vi "test_Bitfile Reload_DMA to Scalar.vi"(8 "error in (no error)":errorcluster, 11 "TestCase in":refnum<class "FPGA Addon Bitfile Reload Unit Tests.lvclass">) -> (0 "error out":errorcluster, 3 "TestCase out":refnum<class "FPGA Addon Bitfile Reload Unit Tests.lvclass">)   [LabVIEW 2020, in "FPGA Addon Bitfile Reload Unit Tests.lvclass"]
uses:
  FPGA Addon Bitfile Reload Unit Tests.lvclass
  APIs/Scripting API/TypeDefs/Output Scalar Data.ctl
  Addon/Addon Shared/Types/FPGA Addon Data Type.ctl
  Addon/Addon Shared/Types/DMA Information.ctl
  Addon/Addon Shared/Types/DMA Settings.ctl
  Addon/Addon Shared/Types/Delacing Scheme.ctl
  Addon/Addon Shared/Types/DMA Acquisition Mode.ctl
  APIs/Scripting API/Public/Bitfile Resources/Import Bitfile Scalars (Instances)/Import Scalars - all.vi
  <vilib>/addons/_JKI Toolkits/VI Tester/TestCase.llb/TestCase.lvclass
  APIs/Scripting API/Scripting API.lvlib
  FPGA Addon Test Class/FPGA Addon Test Class.lvclass
  Addon/Addon System Explorer/FPGA Addon System Explorer.lvlib
  Addon/Addon Shared/FPGA Addon Shared.lvlib
  C:/Program Files (x86)/National Instruments/LabVIEW 2020/vi.lib/addons/_JKI Toolkits/VI Tester/TestCase.llb/TestCase.lvclass
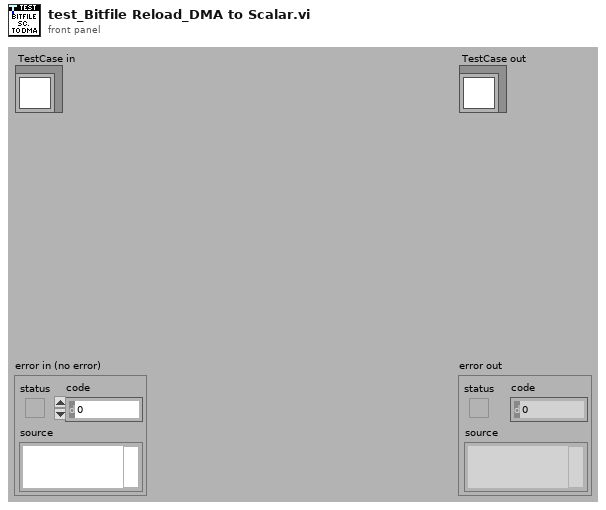
[diagram p1: front panel]
types:
  T1 = typedef "FPGA Addon Shared.lvlib/DMA Information.ctl" = cluster{"Name":string, "Data Type":T2}
  T2 = typedef "FPGA Addon Shared.lvlib/FPGA Addon Data Type.ctl" = enum8{"<Null>", "I8", "I16", "I32", "I64", "U8", "U16", "U32", "U64", "SGL", "Boolean", "Analog PWM In Settings", "Analog PWM In", "Digital PWM In Settings", "Digital PWM In", "Digital PWM Out", "Sine Out", "FXP", "FXP+/-24.5", "FXP+/-16.5", "FXP+/-32.8", "FXP+/-64.32", "FXP+/-16.7", "FXP+/-20.5", "FXP+/-27.5", "FXP+/-32.16", "FXP+16.3", "FXP+18.3", "Digital Static In", "Digital Static Out", "Digital Static In Settings", "Digital WSS Out", "Quad Encoder Settings", "Quad Encoder In", "Group"}
  T3 = typedef "FPGA Addon Shared.lvlib/DMA Settings.ctl" = cluster{"Number of Channels":u8, "Delacing Scheme":T4, "Update Rate":u32, "dt":dbl, "Mode":T5, "Number of Samples":u32, "DMA Host Buffer":u32}
  T4 = typedef "FPGA Addon Shared.lvlib/Delacing Scheme.ctl" = enum8{"Interleaved", "Bitpacked"}
  T5 = typedef "FPGA Addon Shared.lvlib/DMA Acquisition Mode.ctl" = enum8{"Continuous", "Triggered Finite"}
  T6 = typedef "Scripting API.lvlib/Output Scalar Data.ctl" = cluster{"Bitfile Name":string, "SysDef Channel Name":string, "Imported":bool, "Data Type":T2}
  T7 = typedef "Custom Device API.lvlib/Custom Device Item Ref.ctl" = u64
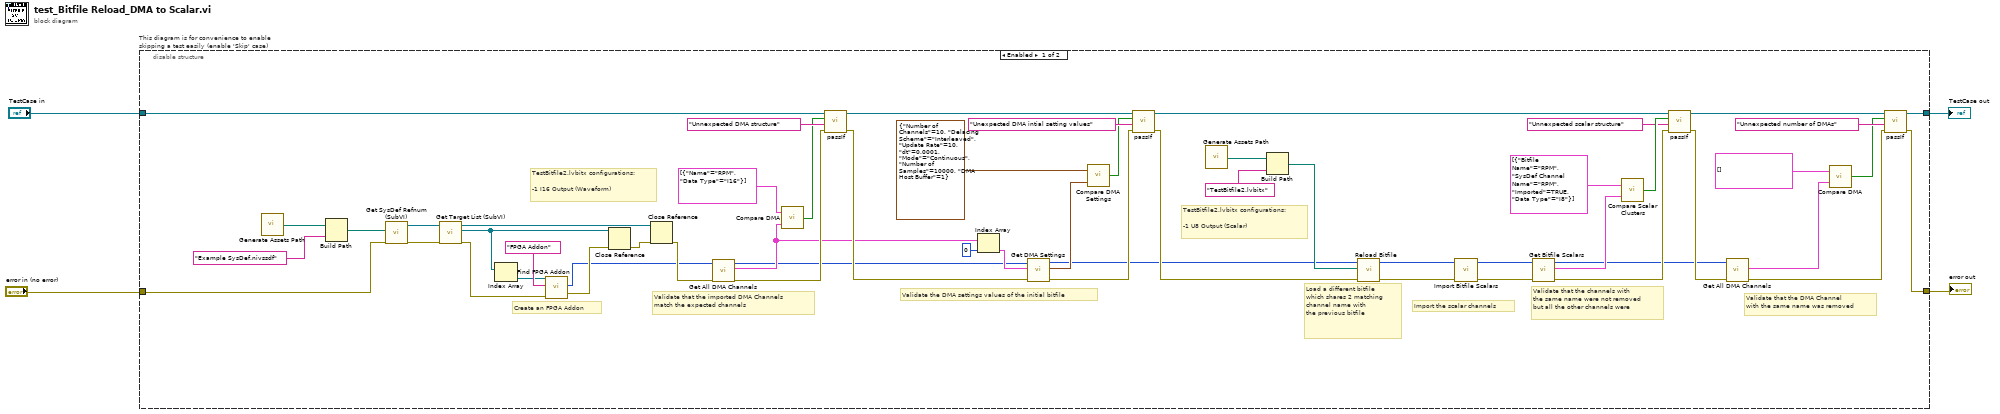
[diagram p0: block diagram]
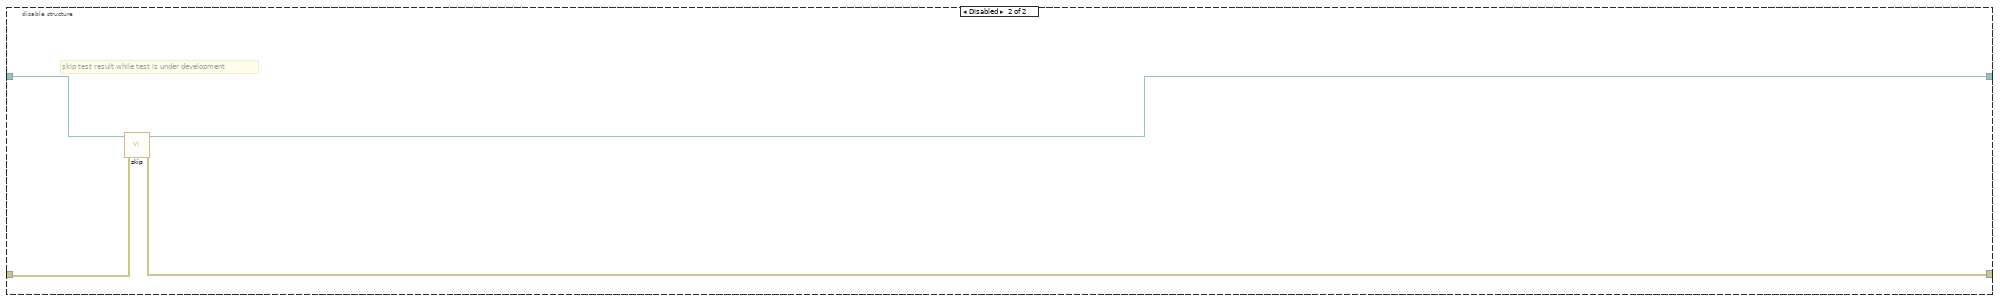
[diagram p2: hidden frame]
diagram:
  n1 = disable-structure "This diagram is for convenience to enable skipping a test easily (enable 'Skip' case)" shown="Enabled" {
    disable-tunnel: "TestCase in" -> [w29 w64]
    disable-tunnel: [w15 w62] -> w1
    disable-tunnel: [w13 w63] -> w3
    disable-tunnel: "error in (no error)" -> [w48 w61]
    frame Enabled {
      # "TestBitfile2.lvbitx configurations:\n\n-1 I16 Output (Waveform)"
      # "Import the scalar channels"
      # "Validate that the DMA Channel \nwith the same name was removed"
      # "Validate the DMA settings values of the initial bitfile"
      # "Validate that the imported DMA Channels \nmatch the expected channels"
      # "Create an FPGA Addon"
      # "TestBitfile2.lvbitx configurations:\n\n-1 U8 Output (Scalar)"
      # "Validate that the channels with \nthe same name were not removed\nbut all the other channels were"
      # "Load a different bitfile\nwhich shares 2 matching\nchannel name with \nthe previous bitfile"
      n2 = call "Generate Assets Path.vi"() -> ("Assets path"=w56:path)
      n3 = Build Path(base path=w56, name or relative path="Example SysDef.nivssdf") -> (appended path=w59:path)
      n4 = call "Get SysDef Refnum (SubVI).vi"("error in (no error)"=w48, "System Definition path"=w59) -> ("error out"=w57:errorcluster, "SysDef Refnum out"=w58:refnum<k24>)  [unwired: 8 in]
      n5 = call "Get Target List (SubVI).vi"("error in (no error)"=w57, "SysDef Refnum in"=w58) -> ("error out"=w26:errorcluster, "Target List Refnums"=w20:refnum<k24>[], "SysDef Refnum out"=w24:refnum<k24>)  [unwired: 7 in]
      n6 = Index Array(array=w20) -> (element=w23:refnum<k24>)  [unwired: 1 in]
      n7 = call "Find FPGA Addon.vi"("error in"=w26, "FPGA addon name"="FPGA Addon", "target in"=w23) -> ("error out"=w44:errorcluster, "FPGA addon refnum out"=w41:T7)  [unwired: 5 in, 2 out]
      n8 = Close Reference(reference=w20, error in (no error)=w44) -> (error out=w46:errorcluster)
      n9 = Close Reference(reference=w24, error in (no error)=w46) -> (error out=w42:errorcluster)
      n10 = call "Get All DMA Channels.vi"("error in (no error)"=w42, "FPGA addon refnum in"=w41) -> ("error out"=w40:errorcluster, "DMA channels out"=w35:T1[], "FPGA addon refnum out"=w30:T7)  [unwired: 7 in]
      n11 = call "Compare DMA.vi"("Target bitfile DMA in"=w35, "Reference bitfile DMA in"=T1[] [{"Name"="RPM", "Data Type"=enum."I16"}] ("DMA channels out")) -> ("Equal ?"=w25:bool)
      n12 = call-dynamic "passIf.vi"("error in (no error)"=w40, "message (\"\")"="Unnexpected DMA structure" ("message (\"\")"), "pass"=w25, "TestCase in"=w29) -> ("error out"=w36:errorcluster, "TestCase out"=w28:refnum<class "FPGA Addon Bitfile Reload Unit Tests.lvclass">)  [unwired: 6 in]
      n13 = Index Array(array=w35, index=0) -> (element=w37:T1)
      n14 = call "Get DMA Settings.vi"("error in (no error)"=w36, "DMA Channel in"=w37, "FPGA addon refnum in"=w30) -> ("error out"=w31:errorcluster, "DMA Settings"=w33:T3, "FPGA addon refnum out"=w9:T7)  [unwired: 6 in]
      n15 = call "Compare DMA Settings.vi"("DMA Settings 2"=w33, "DMA Settings 1"=T3 {"Number of Channels"=10, "Delacing Scheme"=enum."Interleaved", "Update Rate"=10, "dt"=0.0001, "Mode"=enum."Continuous", "Number of Samples"=10000, "DMA Host Buffer"=1} ("DMA Settings")) -> ("equal?"=w21:bool)
      n16 = call-dynamic "passIf.vi"("error in (no error)"=w31, "message (\"\")"="Unexpected DMA intial setting values" ("message (\"\")"), "pass"=w21, "TestCase in"=w28) -> ("error out"=w22:errorcluster, "TestCase out"=w27:refnum<class "FPGA Addon Bitfile Reload Unit Tests.lvclass">)  [unwired: 6 in]
      n17 = call "Generate Assets Path.vi"() -> ("Assets path"=w54:path)
      n18 = Build Path(base path=w54, name or relative path="TestBitfile2.lvbitx") -> (appended path=w53:path)
      n19 = call "Reload Bitfile.vi"("error in (no error)"=w22, "NewVal"=w53, "Item Ref in"=w9) -> ("error out"=w8:errorcluster, "Section Ref out"=w6:T7)  [unwired: 7 in]
      n20 = call-poly "Import Bitfile Scalars.vi"("error in"=w8, "FPGA addon refnum in"=w6) -> ("error out"=w7:errorcluster, "FPGA addon refnum out"=w5:T7)  [unwired: 7 in, 1 out]
      n21 = call "Get Bitfile Scalars.vi"("error in"=w7, "FPGA addon refnum in"=w5) -> ("error out"=w51:errorcluster, "bitfile scalars out"=w52:T6[], "FPGA addon refnum out"=w10:T7)  [unwired: 7 in]
      n22 = call "Compare Scalar Clusters.vi"("Target bitfile scalars in"=w52, "Reference bitfile scalars in"=T6[] [{"Bitfile Name"="RPM", "SysDef Channel Name"="RPM", "Imported"=TRUE, "Data Type"=enum."I8"}] ("imported bitfile scalars out")) -> ("Equal ?"=w50:bool)
      n23 = call-dynamic "passIf.vi"("error in (no error)"=w51, "message (\"\")"="Unnexpected scalar structure" ("message (\"\")"), "pass"=w50, "TestCase in"=w27) -> ("error out"=w18:errorcluster, "TestCase out"=w16:refnum<class "FPGA Addon Bitfile Reload Unit Tests.lvclass">)  [unwired: 6 in]
      n24 = call "Get All DMA Channels.vi"("error in (no error)"=w18, "FPGA addon refnum in"=w10) -> ("error out"=w14:errorcluster, "DMA channels out"=w19:T1[])  [unwired: 7 in, 1 out]
      n25 = call "Compare DMA.vi"("Target bitfile DMA in"=w19, "Reference bitfile DMA in"=T1[] [] ("DMA channels out")) -> ("Equal ?"=w11:bool)
      n26 = call-dynamic "passIf.vi"("error in (no error)"=w14, "message (\"\")"="Unnexpected number of DMAs" ("message (\"\")"), "pass"=w11, "TestCase in"=w16) -> ("error out"=w13:errorcluster, "TestCase out"=w15:refnum<class "FPGA Addon Bitfile Reload Unit Tests.lvclass">)  [unwired: 6 in]
    }
    frame Disabled {
      # "skip test result while test is under development"
      n27 = call <vilib>:"skip.vi"("error in (no error)"=w61, "TestCase in"=w64) -> ("error out"=w63:errorcluster, "TestCase out"=w62:refnum<class "FPGA Addon Bitfile Reload Unit Tests.lvclass">)  [unwired: 8 in]
    }
  }
  "error out" <- w3
  "TestCase out" <- w1
